vi "McP789A-Move-Server v1.00.vi"(6 "Change Counter Position Manually":bool, 7 "error in":errorcluster, 10 "GOTO":dbl format="%.3f") -> (0 "error out":errorcluster={"status"=TRUE, "code"=65, "source"="McP Timeout"}, 1 "ScanStatus":T2, 3 "CurrentPosition":dbl caption="Current Position" format="%.3f")   [LabVIEW 2019]
doc: "McPherson 789A-3 controller Vi to control McPherson 2075 spectrometer through serial port. If running directly, you need to initialize the serial port and the spectrometer. During this process, if the scan velocity returns to be 0, the program is suspended. You need to change the velocity manually to unblock."
uses:
  Sub VIs/McPherson Spectrometer/McPhersonStatus.ctl
  Globals and TypeDefs/Type Definitions.llb/McPherson Status.ctt
  Globals and TypeDefs/gSpectrometer.vi
  Globals and TypeDefs/Global Varibal Control.vi
panel:
  out "McPherson Status":T1
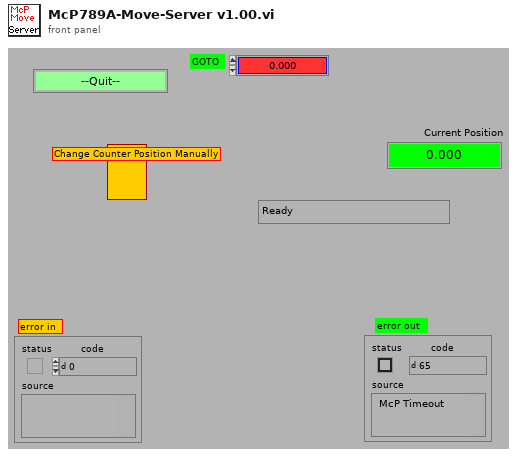
[diagram p1: front panel]
types:
  T1 = typedef "McPherson Status.ctt" = enum8{"--Quit--", "Error", "Initialization", "Standby", "Start Slew", "-Slew", "+Slew", "Slew Done", "Start Scan", "-Slew to Start", "+Slew to Start", "Scanning", "Scan Done", "Scan Pause", "Slew Pause", "Cancel", "Update Z0", "Sleep"}
  T2 = typedef "McPhersonStatus.ctl" = enum16{"Ready", "+Slew", "-Slew", "Slew Done", "Begin Scan", "+Slew to Start", "-Slew to Start", "Scanning", "Scan Done", "Scan Pause", "Slew Pause"}
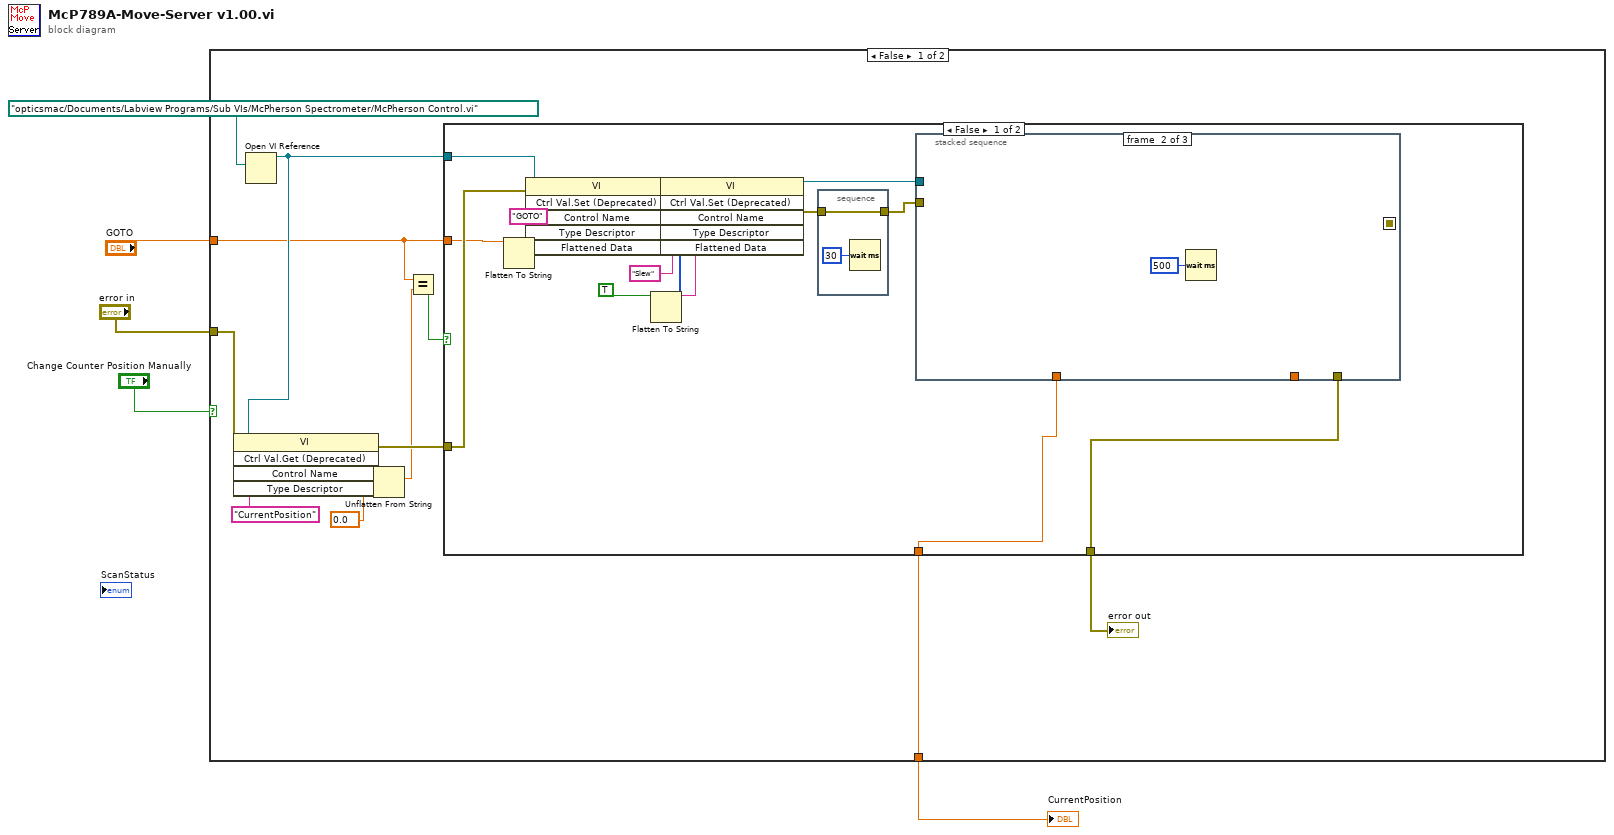
[diagram p0: block diagram]
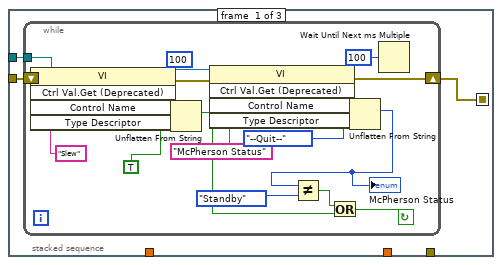
[diagram p2: hidden frame]
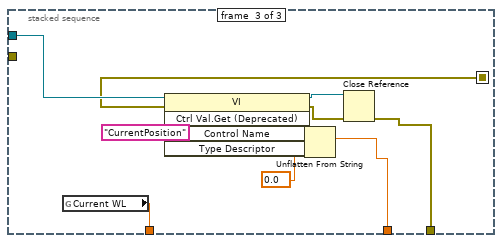
[diagram p3: hidden frame]
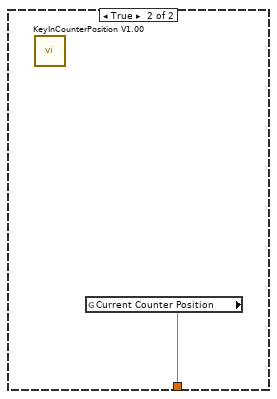
[diagram p5: hidden frame]
diagram:
  n1 = case shown="False" "Change Counter Position Manually" {
    tunnel: [w16 w69] -> w3
    tunnel: "error in" -> [w11 _]
    tunnel: "GOTO" -> [w7 _]
    frame False {
      n2 = Open VI Reference(vi path=path "/opticsmac/Documents/Labview Programs/Sub VIs/McPherson Spectrometer/McPherson Control.vi") -> (vi reference=w10:refnum<vi>)  [unwired: 5 in, 1 out]
      n3 = invoke class="VI" method="Ctrl Val.Get (Deprecated)"(reference=w10, error in=w11, "Control Name"="CurrentPosition") -> (error out=w9:errorcluster, "Get Control Value"=w13:string)  [unwired: 2 in, 3 out]
      n4 = Unflatten From String(type=0.0, binary string=w13) -> (value=w8:dbl)  [unwired: 3 in, 2 out]
      n5 = Equal?(x=w7, y=w8) -> (x = y?=w5:bool)
      n6 = case shown="False" w5 {
        tunnel: [w17 w68] -> w16
        tunnel: w10 -> [w21 _]
        tunnel: w9 -> [w20 w67]
        tunnel: w7 -> [w19 w68]
        tunnel: [w18 w67] -> w6
        frame False {
          n7 = Flatten To String(anything=w19) -> (data string=w31:string, type string=w32:i16[])  [unwired: 3 in, 1 out]
          n8 = invoke class="VI" method="Ctrl Val.Set (Deprecated)"(reference=w21, error in=w20, "Control Name"="GOTO", "Type Descriptor"=w32, "Flattened Data"=w31) -> (reference out=w30:refnum<vi>, error out=w29:errorcluster)  [unwired: 1 in, 4 out]
          n9 = Flatten To String(anything=TRUE ("Wait until done")) -> (data string=w26:string, type string=w27:i16[])  [unwired: 3 in, 1 out]
          n10 = invoke class="VI" method="Ctrl Val.Set (Deprecated)"(reference=w30, error in=w29, "Control Name"="Slew", "Type Descriptor"=w27, "Flattened Data"=w26) -> (reference out=w25:refnum<vi>, error out=w24:errorcluster)  [unwired: 1 in, 4 out]
          n11 = stacked-sequence {
            tunnel: [w65] -> w23
            tunnel: w24 -> [w65]
            frame #0 {
              n12 = Wait (ms)(milliseconds to wait=u32 30) -> ()  [unwired: 1 out]
            }
          }
          n13 = stacked-sequence {
            seq-local: [w34 _ _] -> [_ _ w57]
            tunnel: w25 -> [w36 _ w58]
            tunnel: w23 -> [w35 _ _]
            tunnel: [_ _ w59] -> _
            tunnel: [_ _ w56] -> w18
            tunnel: [_ _ w55] -> w17
            frame #0 {
              n14 = while {
                shift-left: w35 -> [w47]
                shift-right: [w51] -> w34
                tunnel: w36 -> [w46]
                stop <- w42 continue-if-true
                (unwired) u32 100 ("millisecond multiple")
                n15 = invoke class="VI" method="Ctrl Val.Get (Deprecated)"(reference=w46, error in=w47, "Control Name"="Slew") -> (reference out=w45:refnum<vi>, error out=w44:errorcluster, "Get Control Value"=w48:string)  [unwired: 2 in, 2 out]
                n16 = Unflatten From String(type=TRUE ("Wait until done"), binary string=w48) -> (value=w41:bool)  [unwired: 3 in, 2 out]
                n17 = invoke class="VI" method="Ctrl Val.Get (Deprecated)"(reference=w45, error in=w44, "Control Name"="McPherson Status") -> (error out=w51:errorcluster, "Get Control Value"=w52:string)  [unwired: 2 in, 3 out]
                n18 = Unflatten From String(type=McPherson_Status.ctt."--Quit--" ("McPherson Status"), binary string=w52) -> (value=w37:T1)  [unwired: 3 in, 2 out]
                "McPherson Status" <- w37
                n19 = Not Equal?(x=w37, y=McPherson_Status.ctt."Standby" ("McPherson Status")) -> (x != y?=w38:bool)
                n20 = Or(x=w38, y=w41) -> (x .or. y?=w42:bool)
                n21 = Wait Until Next ms Multiple(millisecond multiple=u32 100) -> ()  [unwired: 1 out]
              }
            }
            frame #1 {
              n22 = Wait (ms)(milliseconds to wait=u32 500) -> ()  [unwired: 1 out]
            }
            frame #2 {
              n23 = global read "gSpectrometer.vi" "Current WL"() -> (w55:dbl)
              n24 = invoke class="VI" method="Ctrl Val.Get (Deprecated)"(reference=w58, error in=w57, "Control Name"="CurrentPosition") -> (reference out=w64:refnum<vi>, error out=w63:errorcluster, "Get Control Value"=w61:string)  [unwired: 2 in, 2 out]
              n25 = Unflatten From String(type=0.0, binary string=w61) -> (value=w59:dbl)  [unwired: 3 in, 2 out]
              n26 = Close Reference(reference=w64, error in (no error)=w63) -> (error out=w56:errorcluster)
            }
          }
        }
        frame True {
        }
      }
      "error out" <- w6
    }
    frame True {
      n27 = call "KeyInCounterPosition V1.00.vi"() -> ()  [unwired: 1 in, 2 out]
      n28 = global read "Global Varibal Control.vi" "Current Counter Position"() -> (w69:dbl)
    }
  }
  "CurrentPosition" <- w3
